vi "CanAnalTest.vi"(8 "error in":errorcluster, 11 "Init_Only_F":bool) -> (0 "error out":errorcluster, 1 "CAN sts":bool, 2 "Data out":u8[](array[numeric]), 3 "Res_Pass_T":bool=TRUE, 5 "Config_CANAT_out":refnum<vi>)   [LabVIEW 2017]
uses:
  CAN/CANalystII/PCAN_Driver/ControlCAN.llb/CAN Channel.ctl
  CAN/CANalystII/PCAN_Driver/ControlCAN.llb/DevType.ctl
  CAN/CANalystII/PCAN_Driver/ControlCAN.llb/VCI_INIT_CONFIG.ctl
  CAN/CANalystII/PCAN_Driver/ControlCAN.llb/InitFlag.ctl
  CAN/CANalystII/PCAN_Driver/ControlCAN.llb/Fliter.ctl
  CAN/CANalystII/PCAN_Driver/ControlCAN.llb/Mode.ctl
  CAN/CANalystII/PCAN_Driver/ControlCAN.lvlib
panel:
  out "Config_CANAT":T7 {"DevType" items=["USB-CAN"=3, "USB-CAN2"=4]; "CanIndex" items=["1", "通道2"]; "VCI_INIT_CONFIG"."Fliter" items=["接收所有类型"=3, "只接收标准帧"=4, "只接收扩展帧"=7]; "VCI_INIT_CONFIG"."Mode" items=["正常工作", "自测模式（环回）", "仅侦听模式"]; "VCI_INIT_CONFIG"."InitFlag" items=["使用Flash参数", "使用界面设置参数"]}
  in  "Channel 2":T2 caption="Channel" items=["Channel 1", "Channel 2"]
  in  "CAN Init":bool
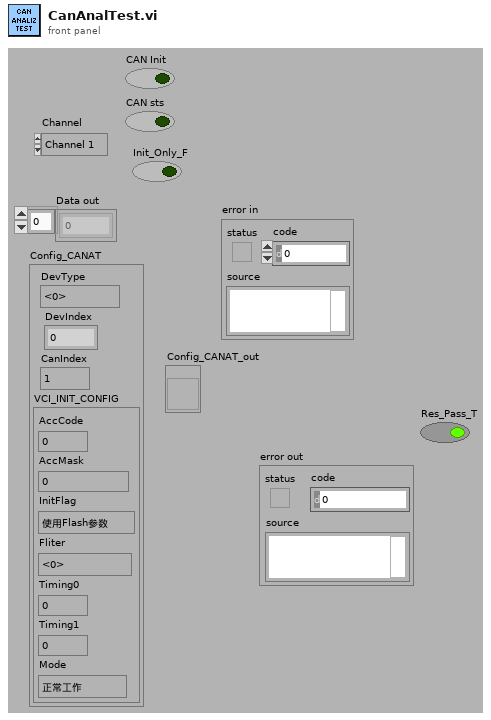
[diagram p1: front panel]
types:
  T1 = typedef "ControlCAN.lvlib/DevType.ctl" = u32
  T2 = typedef "ControlCAN.lvlib/CAN Channel.ctl" = u32
  T3 = typedef "ControlCAN.lvlib/VCI_INIT_CONFIG.ctl" = cluster{"AccCode":u32, "AccMask":u32, "InitFlag":T4, "Fliter":T5, "Timing0":u8, "Timing1":u8, "Mode":T6}
  T4 = typedef "ControlCAN.lvlib/InitFlag.ctl" = u32
  T5 = typedef "ControlCAN.lvlib/Fliter.ctl" = u8
  T6 = typedef "ControlCAN.lvlib/Mode.ctl" = u8
  T7 = cluster{"DevType":T1, "DevIndex":u32, "CanIndex":T2, "VCI_INIT_CONFIG":T3}
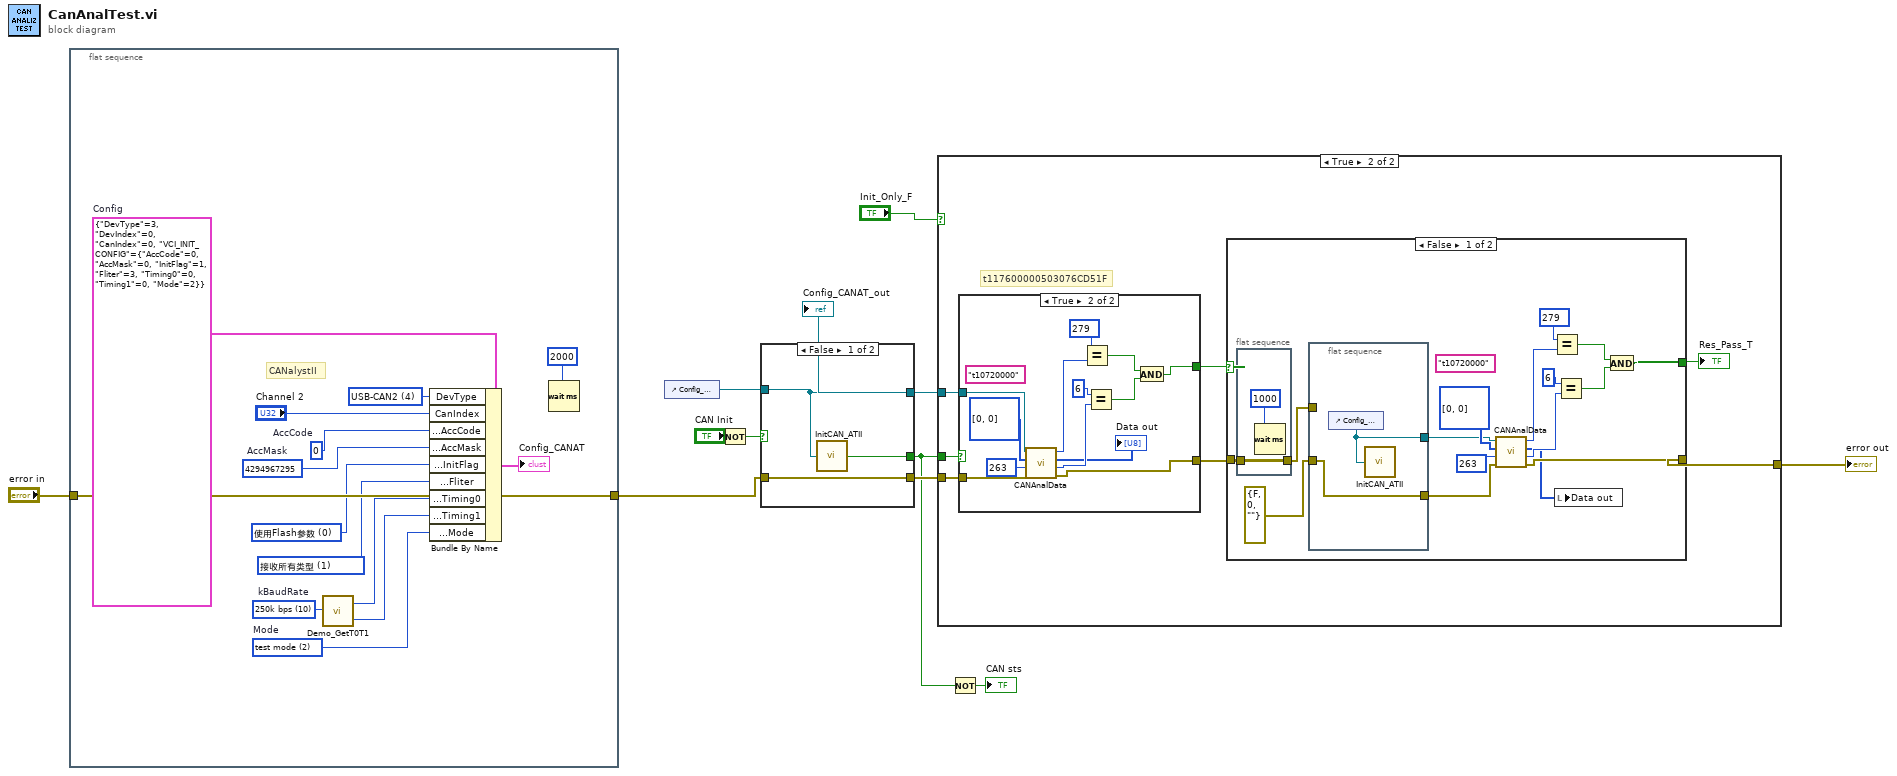
[diagram p0: block diagram]
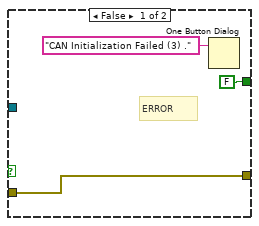
[diagram p4: hidden frame]
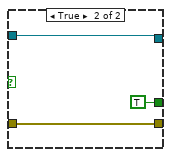
[diagram p5: hidden frame]
diagram:
  n1 = flat-sequence {
    tunnel: "error in" -> [w25]
    tunnel: [w25] -> w4
    frame #0 {
      w16 = u32 4294967295  # AccMask
      w17 = T4 0 items=["使用Flash参数", "使用界面设置参数"] ("InitFlag")
      w22 = T6 2 items=["normal operation", "Listen-only mode", "test mode"]  # Mode
      w18 = T5 1 items=["接收所有类型"=1, "只接收标准帧"=2, "只接收扩展帧"=3] ("Fliter")
      w19 = u8 10 items=["5k bps"=1, "10k bps"=2, "20k bps"=3, "40k bps"=4, "50k bps"=5, "80k bps"=6, "100k bps"=7, "125k bps"=8, "200k bps"=9, "250k bps"=10, "400k bps"=11, "500k bps"=12, "666k bps"=13, "800k bps"=14, "1000k bps"=15, "33.33k bps"=16, "66.66k bps"=17, "83.33k bps"=18]  # kBaudRate
      w15 = u32 0  # AccCode
      w13 = T1 4 items=["USB-CAN"=3, "USB-CAN2"=4] ("DevType")
      w12 = T7 {"DevType"=3, "DevIndex"=0, "CanIndex"=0, "VCI_INIT_CONFIG"={"AccCode"=0, "AccMask"=0, "InitFlag"=1, "Fliter"=3, "Timing0"=0, "Timing1"=0, "Mode"=2}}  # Config
      # "CANalystII"
      n2 = call "Demo_GetT0T1.vi"("kBaudRate"=w19) -> ("Timing0"=w20:u8, "Timing1"=w21:u8)
      n3 = Bundle By Name(cluster=w12, "DevType"=w13, "CanIndex"="Channel 2", "VCI_INIT_CONFIG.AccCode"=w15, "VCI_INIT_CONFIG.AccMask"=w16, "VCI_INIT_CONFIG.InitFlag"=w17, "VCI_INIT_CONFIG.Fliter"=w18, "VCI_INIT_CONFIG.Timing0"=w20, "VCI_INIT_CONFIG.Timing1"=w21, "VCI_INIT_CONFIG.Mode"=w22) -> (→"Config_CANAT":T7)
      n4 = Wait (ms)(milliseconds to wait=u32 2000) -> ()  [unwired: 1 out]
    }
  }
  n5 = control-ref of="Config_CANAT"() -> (w3:refnum<vi>)
  n6 = Not(x="CAN Init") -> (.not. x?=w8:bool)
  n7 = case shown="False" w8 {
    tunnel: [w28 TRUE ("Error F")] -> w9
    tunnel: [w27 w30] -> w10
    tunnel: w4 -> [w27 w30]
    tunnel: w3 -> [w26 w29]
    tunnel: [w26 w29] -> w2
    frame False {
      n8 = call "InitCAN_ATII.vi"("Config"=w26) -> ("Sts"=w28:bool)
    }
    frame True {
    }
  }
  "Config_CANAT_out" <- w2
  n9 = case shown="True" "Init_Only_F" {
    tunnel: w10 -> [w32 w39]
    tunnel: w9 -> [_ w38]
    tunnel: [w32 w34] -> w6
    tunnel: w2 -> [_ w33]
    frame False {
    }
    frame True {
      # "t117600000503076CD51F"
      n10 = case shown="True" w38 {
        tunnel: w39 -> [w64 w77]
        tunnel: [w64 w76] -> w35
        tunnel: [FALSE w66] -> w37
        tunnel: w33 -> [_ w75]
        frame False {
          # "ERROR"
          n11 = One Button Dialog(message="CAN Initialization Failed (3) .") -> ()  [unwired: 1 in, 1 out]
        }
        frame True {
          (unwired) "t10720000" ("write buffer")
          n12 = call "CANAnalData.vi"("error in"=w77, "ID"=u32 263, "Data"=u8[] [0, 0], "Config"=w75) -> ("error out"=w76:errorcluster, "DataLen"=w70:u8, "Data out"=→"Data out":u8[], "ID out"=w71:u32)  [unwired: 3 in, 1 out]
          n13 = Equal?(x=u32 279 ("ID"), y=w71) -> (x = y?=w68:bool)
          n14 = Equal?(x=u8 6, y=w70) -> (x = y?=w67:bool)
          n15 = And(x=w68, y=w67) -> (x .and. y?=w66:bool)
        }
      }
      n16 = case shown="False" w37 {
        selector: w37 -> [_ w61]
        tunnel: [w41 w61] -> w36
        tunnel: w35 -> [w55 w60]
        tunnel: [w49 w60] -> w34
        frame False {
          (unwired) "t10720000" ("write buffer")
          n17 = flat-sequence {
            tunnel: w55 -> [w59]
            tunnel: [w59] -> w53
            frame #0 {
              n18 = Wait (ms)(milliseconds to wait=u32 1000) -> ()  [unwired: 1 out]
            }
          }
          n19 = flat-sequence {
            tunnel: errorcluster {"status"=FALSE, "code"=0, "source"=""} ("error out 4") -> [w57]
            tunnel: [w57] -> w50
            tunnel: w53 -> [_]
            tunnel: [w56] -> w47
            frame #0 {
              n20 = control-ref of="Config_CANAT"() -> (w56:refnum<vi>)
              n21 = call "InitCAN_ATII.vi"("Config"=w56) -> ()  [unwired: 1 out]
            }
          }
          n22 = call "CANAnalData.vi"("error in"=w50, "ID"=u32 263, "Data"=u8[] [0, 0], "Config"=w47) -> ("error out"=w49:errorcluster, "DataLen"=w42:u8, "Data out"=w40:u8[], "ID out"=w46:u32)  [unwired: 3 in, 1 out]
          n23 = Equal?(x=u32 279 ("ID"), y=w46) -> (x = y?=w44:bool)
          n24 = local write "Data out"(w40) -> ()
          n25 = Equal?(x=u8 6, y=w42) -> (x = y?=w52:bool)
          n26 = And(x=w44, y=w52) -> (x .and. y?=w41:bool)
        }
        frame True {
        }
      }
      "Res_Pass_T" <- w36
    }
  }
  "error out" <- w6
  n27 = Not(x=w9) -> (.not. x?=→"CAN sts":bool)
